vi "FTW-CodeGen-GenerateCode.vi"(0 "State In":T2, 5 "XRef":refnum<vi>, 7 "Terms":T1(array[cluster]), 9 "Diagram":refnum<vi>) -> (4 "State Out":T2, 6 "Reply":string[](array[string]), 8 "Generated Code?":bool)   [LabVIEW 2012, in "FTW-JSON-Serialize.xnode"]
uses:
  FTW-JSON-Serialize.xnode
  FTW-CodeGen-State.ctl
panel:
  # "Inputs"
  # "Outputs"
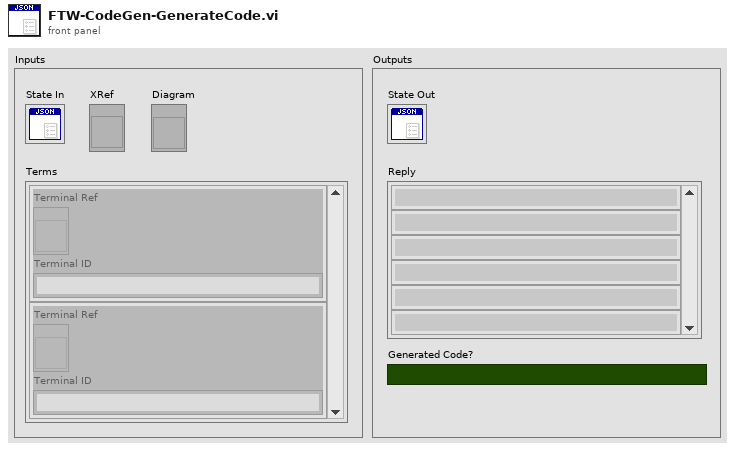
[diagram p1: front panel]
types:
  T1 = cluster{"Terminal Ref":refnum<vi>, "Terminal ID":string}[]
  T2 = typedef "FTW-JSON-Serialize.xnode/FTW-CodeGen-State.ctl" = cluster{"Prototype Filepath":path}
  T3 = typedef "LVPositionTypeDef.ctl" = cluster{"Left":i32, "Top":i32}
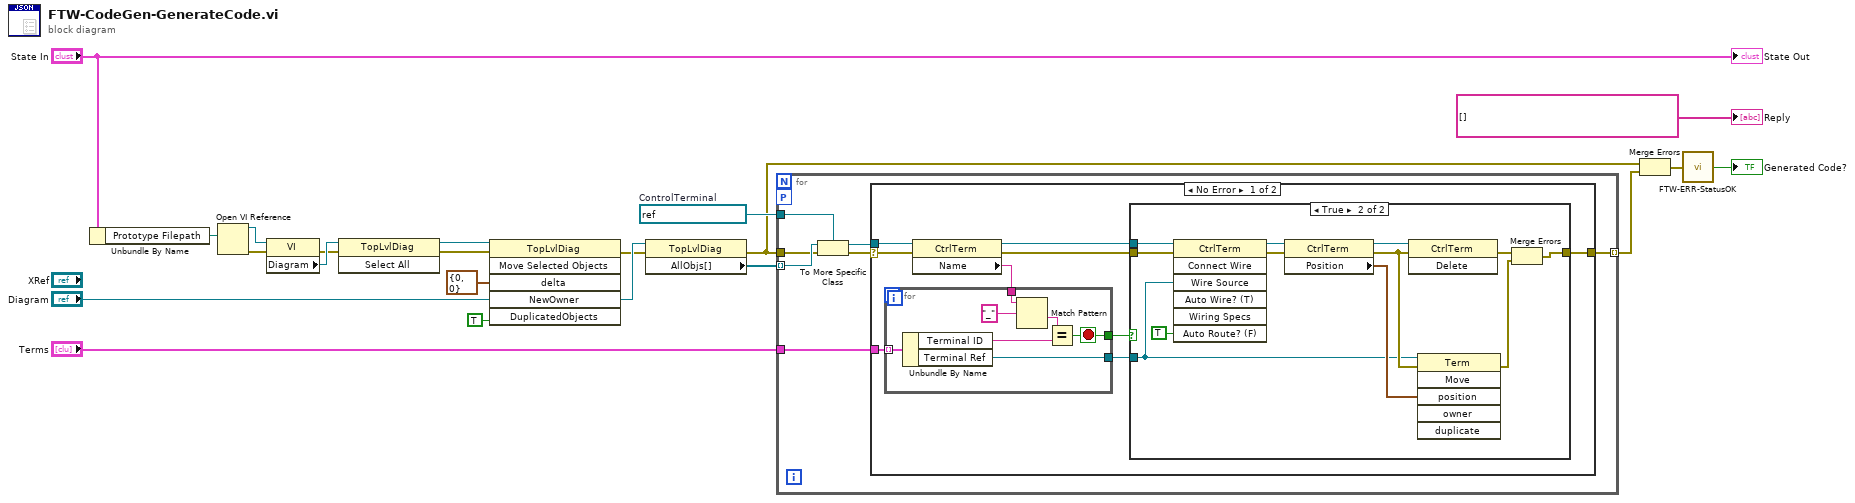
[diagram p0: block diagram]
diagram:
  w14 = refnum<vi> refnum  # ControlTerminal
  n1 = Unbundle By Name("State In") -> ("Prototype Filepath"=w3:path)
  n2 = Open VI Reference(vi path=w3) -> (vi reference=w1:refnum<vi>, error out=w2:errorcluster)  [unwired: 5 in]
  n3 = property class="VI"(reference=w1, error in=w2) -> (error out=w10:errorcluster, "Diagram"=w13:refnum<vi>)  [unwired: 1 out]
  n4 = invoke class="TopLvlDiag" method="Select All"(reference=w13, error in=w10) -> (reference out=w17:refnum<vi>, error out=w16:errorcluster)  [unwired: 1 in, 1 out]
  n5 = invoke class="TopLvlDiag" method="Move Selected Objects"(reference=w17, error in=w16, "delta"=cluster{"X":i32, "Y":i32} {"X"=0, "Y"=0} ("X/Y Delta"), "NewOwner"="Diagram", "DuplicatedObjects"=TRUE ("Duplicate? (F)")) -> (error out=w5:errorcluster)  [unwired: 1 in, 5 out]
  n6 = property class="TopLvlDiag"(reference="Diagram", error in=w5) -> (error out=w11:errorcluster, "AllObjs[]"=w15:refnum<vi>[])  [unwired: 1 out]
  n7 = for {
    tunnel: w15 -> [w27] mode=indexing
    tunnel: w11 -> [w26]
    tunnel: w14 -> [w25]
    tunnel: "Terms" -> [w22]
    tunnel: [w21] -> w12 mode=indexing
    workers-P: _ -> [_]
    n8 = To More Specific Class(target class=w25, reference=w27, error in=w26) -> (specific class reference=w23:refnum<vi>, error out=w24:errorcluster)
    n9 = case shown="No Error" w24 {
      selector: w24 -> [w35 _]
      tunnel: w23 -> [w36 _]
      tunnel: w22 -> [w34 _]
      tunnel: [w29 _] -> w21
      frame No Error {
        n10 = property class="CtrlTerm"(reference=w36, error in=w35) -> (reference out=w31:refnum<vi>, error out=w30:errorcluster, "Name"=w33:string)
        n11 = for {
          tunnel: w34 -> [w56] mode=indexing
          tunnel: w33 -> [w54]
          tunnel: [w55] -> w32
          tunnel: [w50] -> w28
          stop <- w50 stop-if-true
          n12 = Unbundle By Name(w56) -> ("Terminal ID"=w51:string, "Terminal Ref"=w55:refnum<vi>)
          n13 = Match Pattern(string=w54, regular expression="_") -> (after substring=w52:string)  [unwired: 1 in, 3 out]
          n14 = Equal?(x=w52, y=w51) -> (x = y?=w50:bool)
        }
        n15 = case shown="True" w28 {
          tunnel: w32 -> [_ w39]
          tunnel: w31 -> [_ w49]
          tunnel: w30 -> [w37 w48]
          tunnel: [w37 w43] -> w29
          frame False {
          }
          frame True {
            n16 = invoke class="CtrlTerm" method="Connect Wire"(reference=w49, error in=w48, "Wire Source"=w39, "Auto Route? (F)"=TRUE) -> (reference out=w47:refnum<vi>, error out=w45:errorcluster)  [unwired: 3 in, 5 out]
            n17 = property class="CtrlTerm"(reference=w47, error in=w45) -> (reference out=w46:refnum<vi>, error out=w41:errorcluster, "Position"=w40:T3)
            n18 = invoke class="CtrlTerm" method="Delete"(reference=w46, error in=w41) -> (error out=w44:errorcluster)  [unwired: 1 in, 2 out]
            n19 = invoke class="Term" method="Move"(reference=w39, error in=w41, "position"=w40) -> (error out=w42:errorcluster)  [unwired: 3 in, 5 out]
            n20 = Merge Errors(w44, w42) -> (w43:errorcluster)
          }
        }
      }
      frame Error {
      }
    }
  }
  n21 = Merge Errors(w11, w12) -> (w8:errorcluster)
  n22 = call "FTW-ERR-StatusOK.vi"("error to check"=w8) -> ("Status OK?"=→"Generated Code?":bool)
  "State Out" <- "State In"
  "Reply" <- string[] [] ("Reply")
